vi "Show Settings Dialog.vi"(8 "error in (no error)":errorcluster, 11 "Camera Display in":refnum<class "Camera Display.lvclass">) -> (0 "error out":errorcluster, 3 "Camera Display out":refnum<class "Camera Display.lvclass">)   [LabVIEW 2014, in "Camera Display.lvlib" / "Camera Display.lvclass"]
uses:
  Camera Display.lvclass
  Camera Dir Dialog/Camera Dir Dialog/Camera Dir Dialog.lvclass
  Camera Display.lvclass/Camera Display.ctl
  Camera Dir Dialog/Camera Dir Dialog/Camera Dir Dialog.lvclass/Camera Dir Dialog.ctl
  Camera Dir Dialog/Camera Dir Dialog/Write Config Dir.vi
  Camera Dir Dialog/Camera Dir Dialog/Write WorkDir.vi
  <vilib>/ActorFramework/Actor/Actor.lvclass
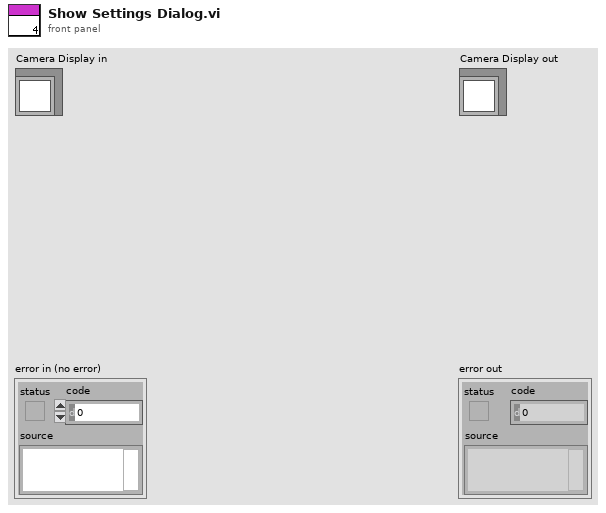
[diagram p1: front panel]
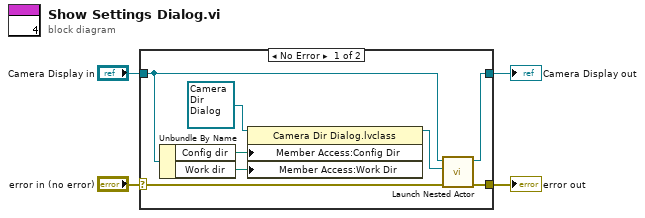
[diagram p0: block diagram]
diagram:
  n1 = case shown="No Error" "error in (no error)" {
    selector: "error in (no error)" -> [w10 w14]
    tunnel: [w9 w14] -> w3
    tunnel: [w12 w13] -> w1
    tunnel: "Camera Display in" -> [w7 w13]
    frame No Error {
      n2 = Unbundle By Name(w7) -> ("Config dir"=w6:path, "Work dir"=w5:path)
      n3 = property class="Camera Dir Dialog.lvclass"(reference=refnum<class "Camera Dir Dialog.lvclass"> refnum ("Camera Dir Dialog.lvlib:Camera Dir Dialog.lvclass"), "Member Access:Config Dir"=w6, "Member Access:Work Dir"=w5) -> (reference out=w8:refnum<class "Camera Dir Dialog.lvclass">)  [unwired: 1 in, 1 out]
      n4 = call <vilib>:"Launch Nested Actor.vi"("error in (no error)"=w10, "Nested Actor"=w8, "Caller Actor in"=w7) -> ("error out"=w9:errorcluster, "Caller Actor out"=w12:refnum<class "Camera Display.lvclass">)  [unwired: 6 in, 1 out]
    }
    frame Error {
    }
  }
  "error out" <- w3
  "Camera Display out" <- w1
